vi "new.vi"(8 "error in (no error)":errorcluster, 11 "data":dbl) -> (0 "error out":errorcluster, 3 "data value reference":refnum<data-value>)   [LabVIEW 2021, in "DoublyNode.lvclass"]
uses:
  DoublyNode.lvclass
  DoublyNode.lvclass/DoublyNode.ctl
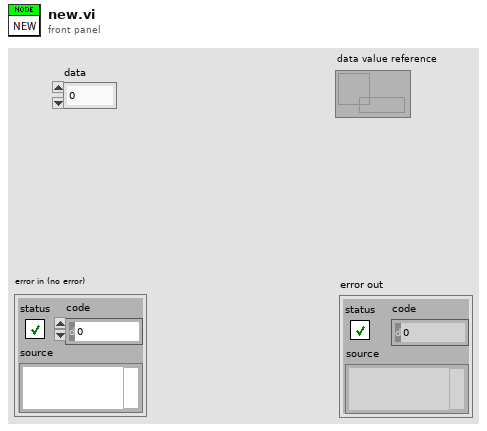
[diagram p1: front panel]
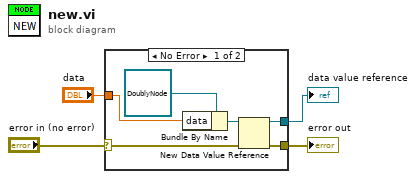
[diagram p0: block diagram]
diagram:
  n1 = case shown="No Error" "error in (no error)" {
    selector: "error in (no error)" -> [w6 w11]
    tunnel: [w5 w11] -> w2
    tunnel: [w8 _] -> w3
    tunnel: "data" -> [w7 _]
    frame No Error {
      n2 = Bundle By Name(cluster=refnum<class "DoublyNode.lvclass"> refnum ("DoublyNode.lvclass"), "data"=w7) -> (w9:refnum<class "DoublyNode.lvclass">)
      n3 = New Data Value Reference(data value=w9, error in=w6) -> (data value reference=w8:refnum<data-value>, error out=w5:errorcluster)
    }
    frame Error {
    }
  }
  "data value reference" <- w3
  "error out" <- w2
